vi "New Vision Server.vi"(2 "error in":errorcluster, 3 "TCP Port":u16) -> (0 "error out":errorcluster, 1 "Vision Server":T1)   [LabVIEW 2016]
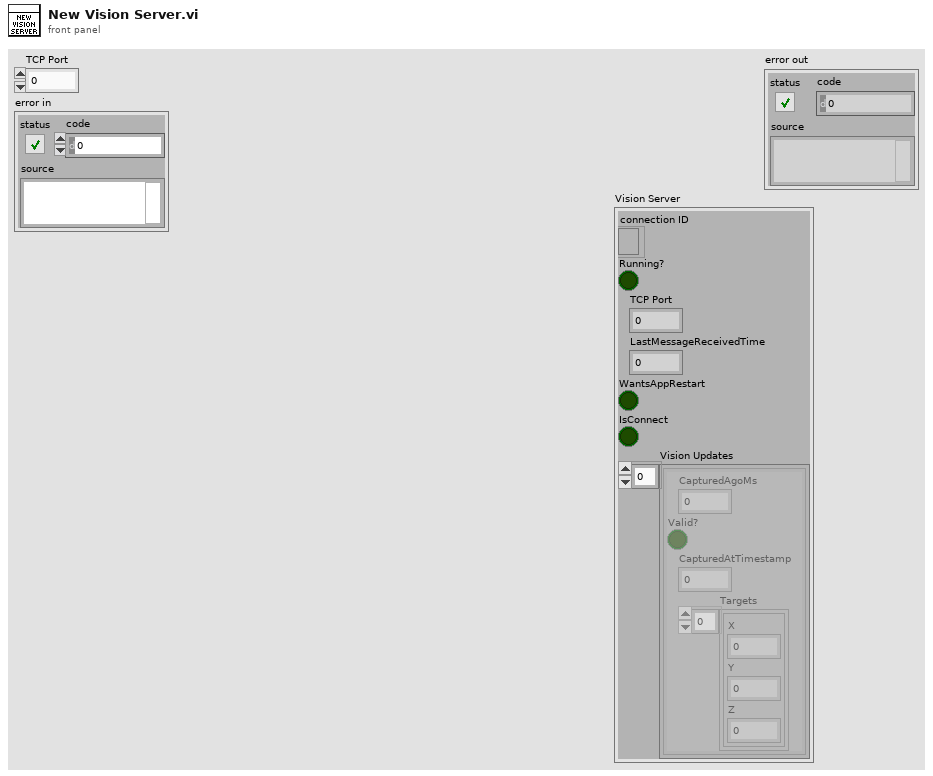
[diagram p1: front panel]
types:
  T1 = cluster{"connection ID":refnum<k5>, "Running?":bool, "TCP Port":u16, "LastMessageReceivedTime":dbl, "WantsAppRestart":bool, "IsConnect":bool, "Vision Updates":cluster{"CapturedAgoMs":i32, "Valid?":bool, "CapturedAtTimestamp":dbl, "Targets":cluster{"X":dbl, "Y":dbl, "Z":dbl}[]}[]}
  T2 = cluster{"CapturedAgoMs":i32, "Valid?":bool, "CapturedAtTimestamp":dbl, "Targets":cluster{"X":dbl, "Y":dbl, "Z":dbl}[]}[]
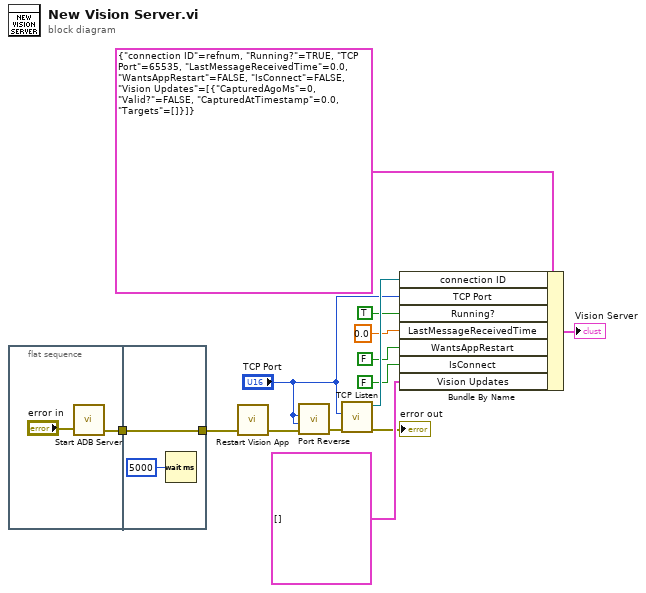
[diagram p0: block diagram]
diagram:
  n1 = flat-sequence {
    tunnel: [w15] -> w1
    tunnel: [w18] -> w3
    tunnel: w1 -> [w18]
    frame #0 {
      n2 = call "Start ADB Server.vi"("error in"="error in") -> ("error out"=w15:errorcluster)  [unwired: 3 in]
    }
    frame #1 {
      n3 = Wait (ms)(milliseconds to wait=u32 5000) -> ()  [unwired: 1 out]
    }
  }
  n4 = call "Restart Vision App.vi"("error in"=w3) -> ("error out"=w2:errorcluster)  [unwired: 1 in, 2 out]
  n5 = call "Port Reverse.vi"("error in"=w2, "local TCP port"="TCP Port", "remote TCP port"="TCP Port") -> ("error out"=w5:errorcluster)  [unwired: 3 in]
  n6 = call <vilib>:"TCP Listen.vi"("error in (no error)"=w5, "port"="TCP Port") -> ("error out"=→"error out":errorcluster, "connection ID"=w13:refnum<k5>)  [unwired: 5 in, 3 out]
  n7 = Bundle By Name(cluster=T1 {"connection ID"=refnum, "Running?"=TRUE, "TCP Port"=65535, "LastMessageReceivedTime"=0.0, "WantsAppRestart"=FALSE, "IsConnect"=FALSE, "Vision Updates"=[{"CapturedAgoMs"=0, "Valid?"=FALSE, "CapturedAtTimestamp"=0.0, "Targets"=[]}]}, "connection ID"=w13, "TCP Port"="TCP Port", "Running?"=TRUE, "LastMessageReceivedTime"=0.0, "WantsAppRestart"=FALSE, "IsConnect"=FALSE, "Vision Updates"=T2 []) -> (→"Vision Server":T1)
